vi "Disconnect from Slave.vi"(8 "error in":errorcluster, 11 "TCP master in":refnum<class "TCP Master.lvclass">) -> (0 "error out":errorcluster, 3 "TCP master out":refnum<class "TCP Master.lvclass">)   [LabVIEW 2021, in "TCP Master.lvclass"]
doc: "Closes the TCP connection stored in the class."
uses:
  TCP Master.lvclass
  D:/my_projects/projects/Algorithms/Labview/21/Modbus_v121c/Network Protocol/Network Master/Network Master.lvclass
  Network Master.lvclass/Network Master.ctl
  Transmission Data Unit/Transmission Data Unit.lvclass
  TCP Master.lvclass/TCP Master.ctl
  Network Master.lvclass
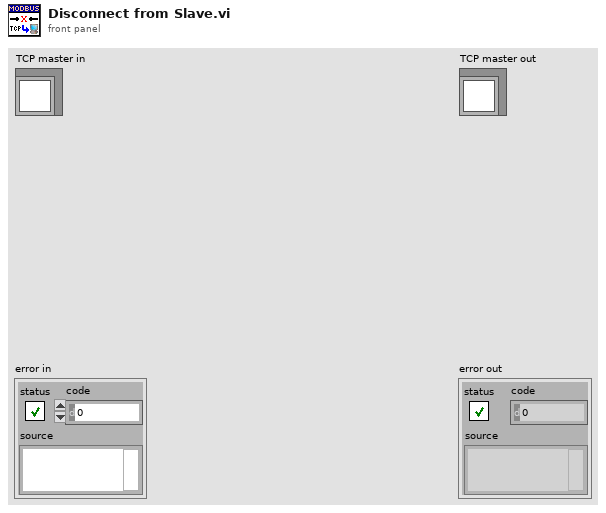
[diagram p1: front panel]
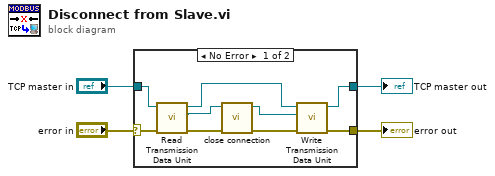
[diagram p0: block diagram]
diagram:
  n1 = case shown="No Error" "error in" {
    selector: "error in" -> [w9 w15]
    tunnel: "TCP master in" -> [w12 w14]
    tunnel: [w11 w15] -> w3
    tunnel: [w10 w14] -> w2
    frame No Error {
      n2 = call "Read Transmission Data Unit.vi"("error in (no error)"=w9, "Network Master in"=w12) -> ("error out"=w8:errorcluster, "Transmission Data Unit"=w6:refnum<class "Transmission Data Unit.lvclass">, "Network Master out"=w13:refnum<class "TCP Master.lvclass">)  [unwired: 7 in]
      n3 = call-dynamic "close connection.vi"("error in"=w8, "transmission data unit in"=w6) -> ("error out"=w7:errorcluster, "transmission data unit out"=w5:refnum<class "Transmission Data Unit.lvclass">)  [unwired: 8 in]
      n4 = call "Write Transmission Data Unit.vi"("error in (no error)"=w7, "Transmission Data Unit"=w5, "Network Master in"=w13) -> ("error out"=w11:errorcluster, "Network Master out"=w10:refnum<class "TCP Master.lvclass">)  [unwired: 7 in]
    }
    frame Error {
    }
  }
  "error out" <- w3
  "TCP master out" <- w2
